vi "UHR-Fleezers Control (host) -Leonardo 04-2018 V4_fish.vi"(0 "Tab Green FB":T5(tab)=enum."Trap Control (RF)") -> ()   [LabVIEW 2014] (continued)
              }
            }
          }
          frame Enabled {
            n955 = call "hamilton_controller.vi"("Open?"=w1537, "valve"=enum16{"A", "B", "C", "D", "ALL"}."A", "action"=T21."MOVE VALVE") -> ()  [unwired: 8 in, 1 out]
          }
        }
      }
      event "Inject Valve B": Value Change {
        n956 = event-data() -> ()  [unwired: 7 out]
        n957 = disable-structure shown="Enabled" {
          disable-tunnel: "Inject Valve B" -> [w1541 w1561]
          frame Disabled {
            n958 = local read "Pump write delay (ms)"() -> (w1543:dbl)
            n959 = flat-sequence {
              tunnel: w1542 -> [w1556]
              tunnel: w1543 -> [w1552]
              tunnel: w1541 -> [_]
              tunnel: w1543 -> [w1558]
              tunnel: w1542 -> [w1559]
              frame #0 {
                n960 = local read "All Pump Parameters"() -> (w1551:T6)
                n961 = Multiply(x=60.0, y="Flush Center Ch Rate (ul/m)") -> (x*y=w1548:dbl)
                n962 = Unbundle By Name(w1551) -> ("Pump 2"=w1557:T33)
                n963 = call "Set pump parameters.vi"("Pump write delay (ms)"=w1552, "Volume (uL)"="Flush Center Ch Volume (uL)", "Rate (uL/h)"=w1548, "Units"=3.0, "Pump #"=2.0, "Pump Parameters In"=w1557, "VISA resource name"=w1556) -> ("Pump Parameters Out"=w1550:T33)  [unwired: 3 in]
                n964 = Bundle By Name(cluster=w1551, "Pump 2"=w1550) -> (w1549:T6)
                n965 = local write "All Pump Parameters"(w1549) -> ()
                n966 = Add(x="Flush Center Ch Volume (uL)", y="Total Volume\nFlushed (uL)") -> (x+y=w1545:dbl)
                n967 = local write "Total Volume\nFlushed (uL)"(w1545) -> ()
              }
              frame #1 {
                n968 = Wait (ms)(milliseconds to wait=w1558) -> ()  [unwired: 1 out]
              }
              frame #2 {
                n969 = call "Write to pump.vi"("string"="start", "VISA resource name"=w1559) -> ()  [unwired: 1 out]
              }
            }
            n970 = local read "Chemyx Syringe Pump Serial Port"() -> (w1542:refnum<visa-resource-name>)
          }
          frame Enabled {
            n971 = call "hamilton_controller.vi"("Open?"=w1561, "valve"=enum16{"A", "B", "C", "D", "ALL"}."B", "action"=T21."MOVE VALVE") -> ()  [unwired: 8 in, 1 out]
          }
        }
      }
      event "Inject Bottom": Value Change {
        n972 = event-data() -> ()  [unwired: 7 out]
        n973 = call "hamilton_controller.vi"("Open?"="Inject Bottom", "valve"=enum16{"A", "B", "C", "D", "ALL"}."C", "action"=T21."MOVE VALVE") -> ()  [unwired: 8 in, 1 out]
      }
      event "Shunt:": Value Change {
        n974 = event-data() -> ()  [unwired: 7 out]
        n975 = call "hamilton_controller.vi"("Open?"="Shunt:", "valve"=enum16{"A", "B", "C", "D", "ALL"}."D", "action"=T21."MOVE VALVE") -> ()  [unwired: 8 in, 1 out]
      }
      event "Flip Green Filter": Value Change {
        n976 = event-data() -> ()  [unwired: 7 out]
        n977 = local write "Flip Green Filter"("Flip Green Filter") -> ()
        n978 = flat-sequence {
          tunnel: w1577 -> [w1582]
          tunnel: w1576 -> [w1581]
          tunnel: [w1579] -> w1574
          tunnel: [w1578] -> w1573
          tunnel: [w1584] -> w1572
          tunnel: w1574 -> [w1584]
          tunnel: [w1583] -> w1571
          tunnel: w1573 -> [w1583]
          tunnel: w1572 -> [w1588]
          tunnel: w1571 -> [w1587]
          tunnel: [w1586] -> w1575
          frame #0 {
            n979 = xnode "Read/Write Control"("FPGA VI Reference In"=w1582, "error in"=w1581, "Green Filter Flipper"=TRUE) -> ("FPGA VI Reference Out"=w1579:T20, "error out"=w1578:errorcluster)
          }
          frame #1 {
            n980 = Wait (ms)(milliseconds to wait=u32 100) -> ()  [unwired: 1 out]
          }
          frame #2 {
            n981 = xnode "Read/Write Control"("FPGA VI Reference In"=w1588, "error in"=w1587, "Green Filter Flipper"=FALSE) -> ("error out"=w1586:errorcluster)  [unwired: 1 out]
          }
        }
      }
      event "Pump 1 contents", "Pump 3 contents": Value Change {
        n982 = event-data() -> ()  [unwired: 7 out]
        n983 = local read "Pump 1 contents"() -> (→"Pump 1 cont disp":string)
        n984 = local read "Pump 3 contents"() -> (→"Pump 3 cont disp":string)
      }
      event "Reset Trap Pos. FB": Value Change {
        n985 = event-data() -> ()  [unwired: 7 out]
        n986 = xnode "Read/Write Control"("FPGA VI Reference In"=w1594, "error in"=w1593, "Trap Pos. FB Reset"="Reset Trap Pos. FB") -> ()  [unwired: 2 out]
      }
      event "Trap Pos. FB ON": Value Change {
        n987 = event-data() -> ()  [unwired: 7 out]
        n988 = xnode "Read/Write Control"("FPGA VI Reference In"=w1609, "error in"=w1608) -> ("FPGA VI Reference Out"=w1606:T20, "BD1 Frequency Out 1"=w1603:u64)  [unwired: 1 out]
        n989 = To Double Precision Float(number=w1603) -> (double precision float=w1602:dbl)
        n990 = Multiply(x=49125000.0, y=6.0) -> (x*y=w1601:dbl)
        n991 = Multiply(x=w1602, y=w1601) -> (x*y=w1599:dbl)
        n992 = Scale By Power Of 2(n=-48, x=w1599) -> (x*2^n=w1598:dbl)
        n993 = Divide(x=w1598, y=1000000.0) -> (x/y=w1595:dbl)
        n994 = flat-sequence {
          tunnel: [w1612] -> w1607
          tunnel: w1606 -> [w1613]
          tunnel: w1603 -> [w1611]
          tunnel: "Trap Pos. FB ON" -> [w1610]
          tunnel: "Trap Pos. FB ON" -> [w1619]
          tunnel: w1607 -> [w1618]
          tunnel: "Trap Pos. FB ON" -> [w1621]
          tunnel: w1595 -> [w1620]
          frame #0 {
            n995 = case shown="False" w1610 {
              tunnel: w1613 -> [w1616 w1617]
              tunnel: [w1615 w1617] -> w1612
              tunnel: w1611 -> [w1614 _]
              frame False {
                n996 = xnode "Read/Write Control"("FPGA VI Reference In"=w1616, "BD 1 Frequency 1"=w1614) -> ("FPGA VI Reference Out"=w1615:T20)  [unwired: 1 in, 1 out]
              }
              frame True {
              }
            }
          }
          frame #1 {
            n997 = xnode "Read/Write Control"("FPGA VI Reference In"=w1618, "Force feedback"=w1619) -> ()  [unwired: 1 in, 2 out]
          }
          frame #2 {
            n998 = case shown="False" w1621 {
              tunnel: w1620 -> [w1624 _]
              frame False {
                n999 = local read "T2 for asymmetric\n(MHz)"() -> (w1622:dbl)
                n1000 = Subtract(x=w1622, y=w1624) -> (x-y=w1623:dbl)
                n1001 = property on="Trap Delta (MHz)" class="DigNum (strict)"("Val(Sgnl)"=w1623) -> ()  [unwired: 2 in, 2 out]
              }
              frame True {
              }
            }
          }
        }
      }
      event "Diff. FB.", "Trap Pos. FB Gains", "Trap Pos. FB Mult Factor", "Trap Pos. FB Offset Factor", "Trap Pos FB Negate Action", "Trap Pos FB Monitor\nT1 or T2", "Negate Diff?": Value Change {
        n1002 = event-data() -> ()  [unwired: 7 out]
        n1003 = xnode "Read/Write Control"("FPGA VI Reference In"=w1635, "error in"=w1634, "Trap pos. FB Range"="Trap Pos. FB Range", "Trap Pos. FB Gains"="Trap Pos. FB Gains", "Trap Pos. FB Mult Factor"="Trap Pos. FB Mult Factor", "Trap Pos. FB Offset Factor"="Trap Pos. FB Offset Factor", "Trap Pos FB Negate Action"="Trap Pos FB Negate Action", "Trap Pos FB Monitor T1 or T2"="Trap Pos FB Monitor\nT1 or T2", "AI1 X Scale"="Trap Pos. AI1 X Pre-scale", "Negate Diff?"="Negate Diff?", "Diff FB Measurement?"="Diff. FB.") -> ()  [unwired: 2 out]
      }
      event "Trap Pos FB SP": Value Change {
        n1004 = event-data() -> ()  [unwired: 7 out]
        n1005 = xnode "Read/Write Control"("FPGA VI Reference In"=w1638, "error in"=w1637, "Trap Pos. FB SP"="Trap Pos FB SP") -> ()  [unwired: 2 out]
        n1006 = disable-structure shown="Disabled" {
          frame Disabled {
            n1007 = local read "Trap X AI1 (DMA)"() -> (w1659:T13)
            n1008 = local read "Trap X (AI1)"() -> (w1660:T1)
            n1009 = local read "Setpoint offset\nCorrection values"() -> (w1653:dbl[])
            n1010 = local read "Trap Delta (MHz)"() -> (w1657:dbl)
            n1011 = local read "B factor"() -> (w1644:dbl)
            n1012 = Unbundle(w1660) -> ("Trap 1"=w1658:fxp<+/-,16,1>, "Trap 2"=w1647:fxp<+/-,16,1>)
            n1013 = Unbundle(w1659) -> ("Set 1"=w1643:fxp<+/-,16,1>, "Set 2"=w1642:fxp<+/-,16,1>)
            n1014 = Negate(x=w1647) -> (-x=w1640:fxp<+/-,17,2>)
            n1015 = Negate(x=w1658) -> (-x=w1641:fxp<+/-,17,2>)
            n1016 = Divide(x=w1657, y=0.1) -> (x/y=w1655:dbl)
            n1017 = Multiply(x=w1642, y=w1644) -> (x*y=w1645:dbl)
            n1018 = Subtract(x=w1643, y=w1645) -> (x-y=w1650:dbl)
            n1019 = To Long Integer(number=w1655) -> (32bit integer=w1654:i32)
            n1020 = Index Array(array=w1653, index=w1654) -> (element=w1649:dbl)
            n1021 = Multiply(x=w1644, y=w1640) -> (x*y=w1646:dbl)
            n1022 = Subtract(x=w1641, y=w1646) -> (x-y=w1652:dbl)
            n1023 = Add(x=w1652, y=w1649) -> (x+y=→"ideal setpoint fpga":dbl)
            n1024 = Add(x=w1650, y=w1649) -> (x+y=→"ideal setpoint avgd":dbl)
          }
          frame Enabled {
          }
        }
        n1025 = disable-structure shown="Enabled" {
          frame Enabled {
          }
          frame Disabled {
            n1026 = local write "B factor"(1.0 ("B factor")) -> ()
          }
        }
      }
      event "Simulate stepping": Value Change {
        n1027 = event-data() -> ()  [unwired: 7 out]
        n1028 = flat-sequence {
          tunnel: w1662 -> [w1665]
          tunnel: [w1664] -> _
          tunnel: w1661 -> [w1663]
          frame #0 {
            n1029 = while {
              tunnel: w1665 -> [w1693]
              tunnel: [w1692] -> w1664 mode=indexing
              tunnel: w1663 -> [w1691]
              i -> [w1677]
              stop <- w1674 stop-if-true
              w1667 = 1000.0
              n1030 = Divide(x="Backtrack probability", y=100) -> (x/y=w1701:dbl)
              n1031 = Random Number (0-1)() -> (number: 0 to 1=w1702:dbl)
              n1032 = Greater?(x=w1702, y=w1701) -> (0:w1700:bool)
              n1033 = Select(t=1, s=w1700, f=-1) -> (s? t:f=w1697:i32)
              n1034 = local read "BD 1 Frequency 2 (MHz)"() -> (w1672:dbl)
              n1035 = Multiply(x=w1697, y="Step size (nm)") -> (x*y=w1695:dbl)
              "Step taken" <- w1695
              n1036 = Divide(x=w1695, y=168.33) -> (x/y=w1670:dbl)
              n1037 = local read "BD 1 Frequency 1 (MHz)"() -> (w1671:dbl)
              n1038 = local read "X RF Frequency Limits (MHz)"() -> (w1690:T16)
              n1039 = local read "Y RF Frequency Limits (MHz)"() -> (w1689:T16)
              n1040 = Subtract(x=w1671, y=w1670) -> (x-y=w1669:dbl)
              n1041 = local write "BD 1 Frequency 1 (MHz)"(w1669) -> ()
              n1042 = local read "BD 2 Frequency 1 (MHz)"() -> (w1687:dbl)
              n1043 = local read "BD 2 Frequency 2 (MHz)"() -> (w1688:dbl)
              n1044 = call "set RF board frequency - interlace.vi"("Board 2 Frequency Limits"=w1689, "Board 1 Frequency Limits"=w1690, "error in"=w1693, "FPGA VI Reference In"=w1691, "Board 2 Frequency 2 (MHz)"=w1688, "Board 2 Frequency 1 (MHz)"=w1687, "Board 1 Frequency 2 (MHz)"=w1672, "Board 1 Frequency 1  (MHz)"=w1669) -> ("error out"=w1692:errorcluster)  [unwired: 2 in, 1 out]
              n1045 = Subtract(x=w1672, y=w1669) -> (x-y=w1686:dbl)
              n1046 = Subtract(x=w1688, y=w1687) -> (x-y=w1685:dbl)
              n1047 = Square(x=w1685) -> (x^2=w1683:dbl)
              n1048 = Square(x=w1686) -> (x^2=w1684:dbl)
              n1049 = Add(x=w1684, y=w1683) -> (x+y=w1682:dbl)
              n1050 = Square Root(x=w1682) -> (sqrt(x)=w1673:dbl)
              n1051 = local write "Trap Delta (MHz)"(w1673) -> ()
              n1052 = property on="Initial delta (MHz)" class="DigNum (strict)"("Val(Sgnl)"=w1673) -> ()  [unwired: 2 in, 2 out]
              n1053 = Multiply(x="Mean dwell time (s)", y=w1667) -> (x*y=w1679:dbl)
              n1054 = case shown="\"Gamma2\"" "Distribution" {
                tunnel: w1679 -> [w1706 w1710 w1713]
                tunnel: [w1706 w1707 w1714] -> w1668
                frame "uniform", Default {
                }
                frame "Exponential" {
                  n1055 = call-poly <vilib>:"Continuous Random.vi"("b"=w1710, "samples"=1) -> ("exp random data"=w1708:dbl[])  [unwired: 8 in, 1 out]
                  n1056 = Index Array(array=w1708) -> (element=w1707:dbl)  [unwired: 1 in]
                }
                frame "Gamma2" {
                  w1711 = 2.0
                  # "Note: the shape and scale\nparameters of the gamma\nare inverted because LabView..."
                  n1057 = Divide(x=w1713, y=w1711) -> (x/y=w1712:dbl)
                  n1058 = call-poly <vilib>:"Continuous Random.vi"("c"=w1712, "b"=w1711, "samples"=1) -> ("gamma random numbers"=w1715:dbl[])  [unwired: 7 in, 1 out]
                  n1059 = Index Array(array=w1715) -> (element=w1714:dbl)  [unwired: 1 in]
                }
              }
              n1060 = Divide(x=w1668, y=w1667) -> (x/y=→"Step duration":dbl)
              n1061 = To Unsigned Long Integer(number=w1668) -> (unsigned 32bit integer=w1680:u32)
              n1062 = Add(x=w1677, y=1) -> (x+y=w1676:i32)
              n1063 = Wait (ms)(milliseconds to wait=w1680) -> ()  [unwired: 1 out]
              n1064 = Equal?(x=w1676, y="Number of steps") -> (x = y?=w1674:bool)
            }
          }
          frame #1 {
            n1065 = local write "Simulate stepping"(FALSE) -> ()
          }
        }
      }
      event "Set SP to Reading": Value Change {
        n1066 = event-data() -> ()  [unwired: 7 out]
        n1067 = local read "Trap Pos FB Monitor\nT1 or T2"() -> (w1725:bool)
        n1068 = local read "Trap X AI1 (DMA)"() -> (w1728:T13)
        n1069 = local read "Trap X (AI1)"() -> (w1731:T1)
        n1070 = Unbundle By Name(w1731) -> ("Trap 1"=w1730:fxp<+/-,16,1>, "Trap 2"=w1729:fxp<+/-,16,1>)
        n1071 = Unbundle By Name(w1728) -> ("Set 1"=w1727:fxp<+/-,16,1>, "Set 2"=w1726:fxp<+/-,16,1>)
        n1072 = Select(t=w1730, s=w1725, f=w1729) -> (s? t:f=w1724:fxp<+/-,16,1>)
        n1073 = Select(t=w1727, s=w1725, f=w1726) -> (s? t:f=w1723:fxp<+/-,16,1>)
        n1074 = Not(x="Set SP Using...") -> (.not. x?=w1718:bool)
        n1075 = Select(t=w1724, s=w1718, f=w1723) -> (s? t:f=w1719:fxp<+/-,16,1>)
        n1076 = xnode "Read/Write Control"("FPGA VI Reference In"=w1721, "error in"=w1720, "Trap Pos. FB SP"=w1719) -> ()  [unwired: 2 out]
        n1077 = local write "Trap Pos FB SP"(w1719) -> ()
      }
      event "Trap Pos. FB Out Scale 2^n": Value Change {
        n1078 = event-data() -> ()  [unwired: 7 out]
        n1079 = Scale By Power Of 2(n="Trap Pos. FB Out Scale 2^n", x=ext 1.0) -> (x*2^n=w1733:ext)
        n1080 = property on="Trap Pos. FB Mult Factor" class="DigNum (strict)"("Val(Sgnl)"=w1733) -> ()  [unwired: 2 in, 2 out]
      }
      event "Trap Pos FB Int Count": Value Change {
        n1081 = event-data() -> ()  [unwired: 7 out]
        n1082 = xnode "Read/Write Control"("FPGA VI Reference In"=w1738, "error in"=w1737, "Trap Pos FB Int Count"="Trap Pos FB Int Count") -> ()  [unwired: 2 out]
      }
      event "Target Force (pN)", "Setpoint offset\nCorrection values", "Raster target force (pN)": Value Change {
        w1747 = 2.0
        n1083 = event-data() -> ()  [unwired: 7 out]
        n1084 = disable-structure "Removed B Factor to improve position feedback - Alex 081418 1of3" shown="Enabled" {
          disable-tunnel: [w1777 fxp<+/-,32,16> 1.0 ("B factor")] -> w1739
          frame Disabled {
            n1085 = local read "B factor"() -> (w1778:dbl)
            n1086 = To Fixed-Point(number=w1778) -> (fixed-point=w1777:fxp<+/-,16,16>)  [unwired: 1 in]
          }
          frame Enabled {
          }
        }
        n1087 = xnode "Read/Write Control"("FPGA VI Reference In"=w1741, "B factor"=w1739) -> ("BD1 Frequency Out 1"=w1768:u64)  [unwired: 1 in, 2 out]
        n1088 = local read "BD 1 Frequency 2 (MHz)"() -> (w1767:dbl)
        n1089 = local read "Target Force (pN)"() -> (w1753:dbl)
        n1090 = To Double Precision Float(number=w1768) -> (double precision float=w1774:dbl)
        n1091 = Multiply(x=49125000.0, y=6.0) -> (x*y=w1773:dbl)
        n1092 = Multiply(x=w1774, y=w1773) -> (x*y=w1771:dbl)
        n1093 = Scale By Power Of 2(n=-48, x=w1771) -> (x*2^n=w1770:dbl)
        n1094 = Divide(x=w1770, y=1000000.0) -> (x/y=w1766:dbl)
        n1095 = Subtract(x=w1767, y=w1766) -> (x-y=w1765:dbl)
        n1096 = local read "T1 kappa_x (pN/nm)"() -> (w1754:dbl)
        n1097 = local read "T1 alpha_x (nm/V)"() -> (w1755:dbl)
        n1098 = local read "Negate offset difference"() -> (w1756:bool)
        n1099 = local read "Offset file step size"() -> (w1764:dbl)
        n1100 = Multiply(x="Raster target force (pN)", y=w1747) -> (x*y=w1746:dbl)
        n1101 = Multiply(x=w1753, y=w1747) -> (x*y=w1752:dbl)
        n1102 = local read "Setpoint offset\nCorrection values"() -> (w1761:dbl[])
        n1103 = Divide(x=w1765, y=w1764) -> (x/y=w1763:dbl)
        n1104 = Select(t=-1, s=w1756, f=1) -> (s? t:f=w1757:i32)
        n1105 = To Long Integer(number=w1763) -> (32bit integer=w1762:i32)
        n1106 = Multiply(x=w1755, y=w1754) -> (x*y=w1745:dbl)
        n1107 = Divide(x=w1752, y=w1745) -> (x/y=w1751:dbl)
        n1108 = Index Array(array=w1761, index=w1762) -> (element=w1760:dbl)
        n1109 = Divide(x=w1746, y=w1745) -> (x/y=w1744:dbl)
        n1110 = Multiply(x=w1757, y=w1760) -> (x*y=w1743:dbl)
        n1111 = Add(x=w1751, y=w1743) -> (x+y=w1750:dbl)
        n1112 = Add(x=w1744, y=w1743) -> (x+y=w1742:dbl)
        n1113 = To Fixed-Point(number=w1742) -> (fixed-point=w1740:fxp<+/-,16,1>)  [unwired: 1 in]
        n1114 = To Fixed-Point(number=w1750) -> (fixed-point=w1749:fxp<+/-,16,1>)  [unwired: 1 in]
        n1115 = property on="Trap Pos FB SP" class="DigNum (strict)"("Val(Sgnl)"=w1749) -> ()  [unwired: 2 in, 2 out]
        n1116 = xnode "Read/Write Control"("FPGA VI Reference In"=w1741, "Raster setpoint"=w1740) -> ()  [unwired: 1 in, 2 out]
      }
      event "Read setpoint correction\nfile": Value Change {
        n1117 = event-data() -> ()  [unwired: 7 out]
        n1118 = local write "Read setpoint correction\nfile"(FALSE) -> ()
        n1119 = Open/Create/Replace File(file path (use dialog)="Setpoint correction\noffset file", operation (0:open)=T24."open", access (0:read/write)=enum16{"read/write", "read-only", "write-only"}."read-only") -> (refnum out=w1805:refnum<file>)  [unwired: 1 in, 4 out]
        n1120 = Deny Access(7:w1805) -> (3:w1803:refnum<file>)  [unwired: 1 in, 2 out]
        n1121 = Read from Binary File(5:0.0, 9:T30."big-endian, network order" ("byte order (0:big-endian, network order)"), 10:-1 ("count (1)"), 11:w1803) -> (2:w1796:dbl[], 3:w1802:refnum<file>)  [unwired: 1 in, 3 out]
        n1122 = Close File(refnum=w1802) -> ()  [unwired: 1 in, 2 out]
        n1123 = Index Array(array=w1796, index=0) -> (element=w1792:dbl)
        n1124 = local write "Offset file step size"(w1792) -> ()
        n1125 = Array Subset(array=w1796, index=3) -> (w1795:dbl[])  [unwired: 1 in]
        n1126 = local read "T1 kappa_x (pN/nm)"() -> (w1790:dbl)
        n1127 = local read "T1 alpha_x (nm/V)"() -> (w1791:dbl)
        n1128 = local read "T2 alpha_x (nm/V)"() -> (w1789:dbl)
        n1129 = local read "T2 kappa_x (pN/nm)"() -> (w1788:dbl)
        n1130 = Decimate 1D Array(w1795) -> (w1784:dbl[], w1785:dbl[])  [unwired: 1 out]
        n1131 = local read "Offset Values"() -> (w1794:T14)
        n1132 = Multiply(x=w1791, y=w1790) -> (x*y=w1786:dbl)
        n1133 = Multiply(x=w1789, y=w1788) -> (x*y=w1787:dbl)
        n1134 = Bundle By Name(cluster=w1794, "Trap 1X offset"=w1784, "Trap 2X offset"=w1785) -> (w1793:T14)
        n1135 = Divide(x=w1787, y=w1786) -> (x/y=w1781:dbl)
        n1136 = disable-structure "Removed B Factor to better position FB - Alex 081418 3of3" shown="Enabled" {
          disable-tunnel: w1781 -> [w1809 _]
          disable-tunnel: [w1809 1.0] -> w1780
          frame Disabled {
          }
          frame Enabled {
          }
        }
        n1137 = Multiply(x=w1785, y=w1780) -> (x*y=w1783:dbl[])
        n1138 = local write "Offset Values"(w1793) -> ()
        n1139 = Subtract(x=w1784, y=w1783) -> (x-y=w1782:dbl[])
        n1140 = property on="B factor" class="DigNum (strict)"("Val(Sgnl)"=w1780) -> ()  [unwired: 2 in, 2 out]
        n1141 = property on="Setpoint offset\nCorrection values" class="Arr (strict)"("Val(Sgnl)"=w1782) -> ()  [unwired: 2 in, 2 out]
      }
      event "MCL Tracking": Value Change {
        n1142 = event-data() -> ()  [unwired: 7 out]
        n1143 = case shown="True" "MCL Tracking" {
          frame False {
            n1144 = local read "Current MCL (V)"() -> (w1812:dbl)
            n1145 = local write "AO2"(w1812) -> ()
          }
          frame True {
            n1146 = local read "BD 1 Frequency 1 (MHz)"() -> (→"Zero T1 position":dbl)
            n1147 = local read "AO2"() -> (→"Zero MCL x position":dbl)
          }
        }
      }
      event "Scale intensities": Value Change {
        n1148 = event-data() -> ()  [unwired: 7 out]
        n1149 = local read "Trap Intensity\nSetpoints (V)"() -> (w1818:cluster{"Set 1":dbl, "Set 2":dbl})
        n1150 = local read "T1 kappa_x (pN/nm)"() -> (w1824:dbl)
        n1151 = local read "T2 kappa_x (pN/nm)"() -> (w1823:dbl)
        n1152 = Unbundle By Name(w1818) -> ("Set 1"=w1820:dbl, "Set 2"=w1819:dbl)
        n1153 = case shown="True" "Scale intensities" {
          tunnel: "Scale factor" -> [w1834 w1846]
          tunnel: "Scale factor" -> [w1829 w1839]
          tunnel: w1824 -> [w1836 w1845]
          tunnel: w1823 -> [w1835 w1844]
          tunnel: [w1832 w1843] -> w1822
          tunnel: [w1833 w1842] -> w1821
          tunnel: w1820 -> [w1831 w1841]
          tunnel: w1819 -> [w1830 w1840]
          tunnel: [w1828 w1838] -> w1817
          tunnel: [w1827 w1837] -> w1816
          frame False {
            n1154 = Divide(x=w1836, y=w1829) -> (x/y=w1832:dbl)
            n1155 = Divide(x=w1835, y=w1834) -> (x/y=w1833:dbl)
            n1156 = Divide(x=w1831, y=w1829) -> (x/y=w1828:dbl)
            n1157 = Divide(x=w1830, y=w1829) -> (x/y=w1827:dbl)
          }
          frame True {
            n1158 = Multiply(x=w1841, y=w1839) -> (x*y=w1838:dbl)
            n1159 = Multiply(x=w1840, y=w1839) -> (x*y=w1837:dbl)
            n1160 = Multiply(x=w1845, y=w1839) -> (x*y=w1843:dbl)
            n1161 = Multiply(x=w1846, y=w1844) -> (x*y=w1842:dbl)
          }
        }
        n1162 = local write "T2 kappa_x (pN/nm)"(w1821) -> ()
        n1163 = local write "T1 kappa_x (pN/nm)"(w1822) -> ()
        n1164 = Bundle By Name(cluster=w1818, "Set 1"=w1817, "Set 2"=w1816) -> (w1815:cluster{"Set 1":dbl, "Set 2":dbl})
        n1165 = property on="Trap Intensity\nSetpoints (V)" class="Clust (strict)"("Val(Sgnl)"=w1815) -> ()  [unwired: 2 in, 2 out]
      }
    }
    "error out 2" <- w773
    n1166 = node-c288() -> ()  [unwired: 1 in, 1 out]
  }
  n1167 = node-c288() -> (w104:T25)  [unwired: 4 in]
  n1168 = timed-loop "Run Scripts, including: stage motion" {
    timing: w104 -> [_]
    timing-out: [_] -> w103
    tunnel: w62 -> [_]
    stop <- w1848 stop-if-true
    n1169 = node-c288() -> ()  [unwired: 1 in, 1 out]
    n1170 = event shown="[0] \"Move Cap. 1 (DNA Top)\": Value Change" {
      selector: _ -> [_ _ _ _ _ _ _ _ _ _ _ _]
      dyn-events: _ -> [_ _ _ _ _ _ _ _ _ _ _ _]
      timeout: 50 -> [_ _ _ _ _ _ _ _ _ _ _ _]
      tunnel: ["Move Cap. 1 (DNA Top)" _ "Cal/Data Acq. Spot" "Dump Beads" "Dip for Protein" _ "Got ADig bead" "Got DNA bead" "Take Stepping Data" _ "Take Detection Laser\nImage" _] -> _
      tunnel: [_ _ _ _ _ _ _ _ _ _ _ w2058] -> w1848
      event "Move Cap. 1 (DNA Top)": Value Change {
        n1171 = event-data() -> ()  [unwired: 1 in, 5 out]
        n1172 = local write "Move Cap. 1 (DNA Top)"(FALSE ("Move Cap. 1 (DNA Right)")) -> ()
        n1173 = flat-sequence {
          tunnel: "Cap 1 Samp Flow ON" -> [w1854]
          frame #0 {
            n1174 = local write "Stage Moving"(FALSE ("Stage Moving")) -> ()
            n1175 = case "stop flow" shown="True" w1854 {
              frame False {
              }
              frame True {
                n1176 = call "hamilton_controller.vi"("Open?"=FALSE, "valve"=enum16{"A", "B", "C", "D", "ALL"}."C", "action"=T21."MOVE VALVE") -> ()  [unwired: 8 in, 1 out]
              }
            }
            n1177 = case shown="True" TRUE {
              tunnel: "Cap 1 T ON" -> [w1863 w1864]
              frame False {
                n1178 = property on="Trap 1 (ON/OFF)" class="Bool (strict)"("Val(Sgnl)"=w1863) -> ()  [unwired: 2 in, 2 out]
              }
              frame True {
                n1179 = property on="Trap 2 (ON/OFF)" class="Bool (strict)"("Val(Sgnl)"=w1864) -> ()  [unwired: 2 in, 2 out]
              }
            }
            n1180 = call <vilib>:"Beep.vi"() -> ()  [unwired: 3 in, 9 out]
            n1181 = case shown="True" "Cap 1 Flow ON" {
              frame False {
              }
              frame True {
                n1182 = property on="Main:" class="Bool (strict)"("Val(Sgnl)"=TRUE ("Value (Signaling)")) -> ()  [unwired: 2 in, 2 out]
              }
            }
          }
        }
      }
      event Timeout {
        n1183 = event-data() -> ()  [unwired: 1 in, 2 out]
      }
      event "Cal/Data Acq. Spot": Value Change {
        # "wait for calibration file\nto be written"
        # "signal save cal true\nthis tells the data \nacquisition loop to\nstart sending the data\nto a calibration file"
        # "separate traps to\nthe desired trap delta"
        # "move stage to data acquisition spot"
        # "CHANGE FISH FOR TETHER BACK\nTO TRUE VALUE HERE."
        n1184 = event-data() -> ()  [unwired: 1 in, 5 out]
        n1185 = flat-sequence {
          tunnel: ["Cal @ (MHz)"] -> w1865
          tunnel: w1865 -> [w1877]
          tunnel: w1865 -> [w1898]
          frame #0 {
            n1186 = property on="Trap Delta (MHz)" class="DigNum (strict)"("Val(Sgnl)"="Cal @ (MHz)") -> ()  [unwired: 2 in, 2 out]
            n1187 = call <vilib>:"Beep.vi"() -> ()  [unwired: 3 in, 9 out]
          }
          frame #1 {
            n1188 = local read "Scale intensities"() -> (w1869:bool)
            n1189 = case shown="True" w1869 {
              frame False {
              }
              frame True {
                n1190 = property on="Scale intensities" class="Bool (strict)"("Val(Sgnl)"=FALSE ("Value (Signaling)")) -> ()  [unwired: 2 in, 2 out]
              }
            }
          }
          frame #2 {
            n1191 = Wait (ms)(milliseconds to wait=u32 500) -> ()  [unwired: 1 out]
          }
          frame #3 {
            n1192 = property on="Save Calibration" class="Bool (strict)"("Val(Sgnl)"=TRUE ("Value (Signaling)")) -> ()  [unwired: 2 in, 2 out]
          }
          frame #4 {
            n1193 = Wait (ms)(milliseconds to wait=u32 4000) -> ()  [unwired: 1 out]
          }
          frame #5 {
            n1194 = while {
              stop <- w1874 stop-if-true
              n1195 = local read "Saving..."() -> (w1875:bool)
              n1196 = Wait (ms)(milliseconds to wait=u32 100) -> ()  [unwired: 1 out]
              n1197 = Not(x=w1875) -> (.not. x?=w1874:bool)
            }
          }
          frame #6 {
            n1198 = case shown="True" "W/ Offset 1" {
              tunnel: w1877 -> [_ w1879]
              frame False {
              }
              frame True {
                n1199 = stacked-sequence {
                  tunnel: w1879 -> [_ _ _ _ _ _ _ w1896]
                  frame #0 {
                    n1200 = Replace Array Subset(array=u32[] [0] ("Index Values"), new element="Offset 1 Set", index=0) -> (w1880:u32[])
                    n1201 = property on="Saved AOD Raster Scan Parameter Sets" class="Arr (strict)"("Index Values"=w1880) -> ()  [unwired: 2 in, 2 out]
                    n1202 = property on="Trap Delta (MHz)" class="DigNum (strict)"("Val(Sgnl)"="Offset 1 Start (MHz)") -> ()  [unwired: 2 in, 2 out]
                  }
                  frame #1 {
                    n1203 = Wait (ms)(milliseconds to wait=u32 200) -> ()  [unwired: 1 out]
                  }
                  frame #2 {
                    n1204 = property on="Load parameters" class="Bool (strict)"("Val(Sgnl)"=TRUE ("Value (Signaling)")) -> ()  [unwired: 2 in, 2 out]
                  }
                  frame #3 {
                    n1205 = Wait (ms)(milliseconds to wait=u32 200) -> ()  [unwired: 1 out]
                  }
                  frame #4 {
                    n1206 = property on="Trap Raster Scan" class="Bool (strict)"("Val(Sgnl)"=TRUE ("Value (Signaling)")) -> ()  [unwired: 2 in, 2 out]
                  }
                  frame #5 {
                    n1207 = Wait (ms)(milliseconds to wait=u32 2000) -> ()  [unwired: 1 out]
                  }
                  frame #6 {
                    n1208 = while {
                      stop <- w1893 stop-if-true
                      n1209 = local read "Raster Scanning..."() -> (w1895:bool)
                      n1210 = local read "Saving..."() -> (w1891:bool)
                      n1211 = Wait (ms)(milliseconds to wait=u32 100) -> ()  [unwired: 1 out]
                      n1212 = Not(x=w1891) -> (.not. x?=w1890:bool)
                      n1213 = Not(x=w1895) -> (.not. x?=w1892:bool)
                      n1214 = And(x=w1892, y=w1890) -> (x .and. y?=w1893:bool)
                    }
                  }
                  frame #7 {
                    n1215 = property on="Trap Delta (MHz)" class="DigNum (strict)"("Val(Sgnl)"=w1896) -> ()  [unwired: 2 in, 2 out]
                  }
                }
              }
            }
          }
          frame #7 {
            n1216 = local read "Save ave N"() -> (w1897:dbl)
            n1217 = case shown="True" "W/ Offset 2" {
              tunnel: w1898 -> [_ w1904]
              tunnel: w1897 -> [_ w1903]
              frame False {
                n1218 = Multiply(x="Cal read wait (s)", y=u32 1000 ("milliseconds to wait")) -> (x*y=w1901:u32)
                n1219 = Wait (ms)(milliseconds to wait=w1901) -> ()  [unwired: 1 out]
              }
              frame True {
                n1220 = stacked-sequence {
                  tunnel: w1904 -> [_ _ _ _ _ _ _ _ _ w1925 _ _]
                  tunnel: w1903 -> [_ _ _ _ _ _ _ _ _ w1923 _ _]
                  frame #0 {
                    n1221 = property on="Save ave N" class="DigNum (strict)"("Val(Sgnl)"=1.0 ("Value (Signaling)")) -> ()  [unwired: 2 in, 2 out]
                  }
                  frame #1 {
                    n1222 = Wait (ms)(milliseconds to wait=u32 500) -> ()  [unwired: 1 out]
                  }
                  frame #2 {
                    n1223 = property on="Trap Delta (MHz)" class="DigNum (strict)"("Val(Sgnl)"="Offset 2 Start (MHz)") -> ()  [unwired: 2 in, 2 out]
                    n1224 = Replace Array Subset(array=u32[] [0] ("Index Values"), new element="Offset 2 Set", index=0) -> (w1909:u32[])
                    n1225 = property on="Saved AOD Raster Scan Parameter Sets" class="Arr (strict)"("Index Values"=w1909) -> ()  [unwired: 2 in, 2 out]
                  }
                  frame #3 {
                    n1226 = Wait (ms)(milliseconds to wait=u32 500) -> ()  [unwired: 1 out]
                  }
                  frame #4 {
                    n1227 = property on="Load parameters" class="Bool (strict)"("Val(Sgnl)"=TRUE ("Value (Signaling)")) -> ()  [unwired: 2 in, 2 out]
                  }
                  frame #5 {
                    n1228 = Wait (ms)(milliseconds to wait=u32 500) -> ()  [unwired: 1 out]
                  }
                  frame #6 {
                    n1229 = property on="Trap Raster Scan" class="Bool (strict)"("Val(Sgnl)"=TRUE ("Value (Signaling)")) -> ()  [unwired: 2 in, 2 out]
                  }
                  frame #7 {
                    n1230 = Wait (ms)(milliseconds to wait=u32 2000) -> ()  [unwired: 1 out]
                  }
                  frame #8 {
                    n1231 = while {
                      stop <- w1918 stop-if-true
                      n1232 = local read "Raster Scanning..."() -> (w1921:bool)
                      n1233 = local read "Saving..."() -> (w1919:bool)
                      n1234 = Wait (ms)(milliseconds to wait=u32 100) -> ()  [unwired: 1 out]
                      n1235 = Not(x=w1919) -> (.not. x?=w1917:bool)
                      n1236 = Not(x=w1921) -> (.not. x?=w1920:bool)
                      n1237 = And(x=w1920, y=w1917) -> (x .and. y?=w1918:bool)
                    }
                  }
                  frame #9 {
                    n1238 = property on="Trap Delta (MHz)" class="DigNum (strict)"("Val(Sgnl)"=w1925) -> ()  [unwired: 2 in, 2 out]
                    n1239 = property on="Saved AOD Raster Scan Parameter Sets" class="Arr (strict)"("Index Values"=u32[] [0]) -> ()  [unwired: 2 in, 2 out]
                    n1240 = property on="Save ave N" class="DigNum (strict)"("Val(Sgnl)"=w1923) -> ()  [unwired: 2 in, 2 out]
                  }
                  frame #10 {
                    n1241 = Wait (ms)(milliseconds to wait=u32 500) -> ()  [unwired: 1 out]
                  }
                  frame #11 {
                    n1242 = property on="Load parameters" class="Bool (strict)"("Val(Sgnl)"=TRUE ("Value (Signaling)")) -> ()  [unwired: 2 in, 2 out]
                  }
                }
              }
            }
          }
          frame #8 {
            n1243 = property on="Read Cal" class="Bool (strict)"("Val(Sgnl)"=TRUE ("Value (Signaling)")) -> ()  [unwired: 2 in, 2 out]
          }
          frame #9 {
            n1244 = Wait (ms)(milliseconds to wait=u32 500) -> ()  [unwired: 1 out]
          }
          frame #10 {
            n1245 = property on="Fish for Tether" class="Bool (strict)"("Val(Sgnl)"=FALSE ("Value (Signaling)")) -> ()  [unwired: 2 in, 2 out]
          }
        }
        n1246 = local write "Cal/Data Acq. Spot"(FALSE ("Cal/Data Acq. Spot")) -> ()
      }
      event "Dump Beads": Value Change {
        # "SCRIPT TO REMOVE BOTH BEADS FROM THE TRAPS. TURNS ON LIGHT WHICH INDICATES THAT STAGE IS MOVING. THEN STOPS SAVING DATA. \nSETS Sample Channel Flow TO TRUE. STOPS INTERLACING GREEN FLUORESCENCE. TURNS OFF Tether INDICATOR BECAUSE WE ARE THROWING IT\nAWAY. SHUTS OFF TRAP POSITION FEEDBACK."
        n1247 = event-data() -> ()  [unwired: 1 in, 5 out]
        n1248 = flat-sequence {
          frame #0 {
            w1932 = FALSE ("Fl. Triggered...")
            w1933 = TRUE ("Stage Moving")
            n1249 = local read "Saving..."() -> (w1934:bool)
            n1250 = local write "Fl. Triggered..."(w1932) -> ()
            n1251 = local write "Stage Moving"(w1933) -> ()
            n1252 = local write "Tether"(w1932) -> ()
            n1253 = property on="Green Laser ON/Interlacing" class="Bool (strict)"("Val(Sgnl)"=w1932) -> ()  [unwired: 2 in, 2 out]
            n1254 = property on="Trap Pos. FB ON" class="Bool (strict)"("Val(Sgnl)"=w1932) -> ()  [unwired: 2 in, 2 out]
            n1255 = property on="Inject Bottom" class="Bool (strict)"("Val(Sgnl)"=w1933) -> ()  [unwired: 2 in, 2 out]
            n1256 = local write "Stop Saving"(w1934) -> ()
          }
          frame #1 {
            w1935 = FALSE ("Value (Signaling)")
            # "TURNS TRAPS OFF SO THAT\nBEADS REMAIN AT DUMP \nBEADS POSITION"
            n1257 = property on="Trap 1 (ON/OFF)" class="Bool (strict)"("Val(Sgnl)"=w1935) -> ()  [unwired: 2 in, 2 out]
            n1258 = property on="Trap 2 (ON/OFF)" class="Bool (strict)"("Val(Sgnl)"=w1935) -> ()  [unwired: 2 in, 2 out]
            n1259 = call <vilib>:"Beep.vi"() -> ()  [unwired: 3 in, 9 out]
          }
          frame #2 {
            n1260 = property on="Goto Bottom (F7)" class="Bool"("Val(Sgnl)"=TRUE ("Value (Signaling)")) -> ()  [unwired: 2 in, 2 out]
          }
          frame #3 {
            n1261 = Wait (ms)(milliseconds to wait=u32 8000) -> ()  [unwired: 1 out]
          }
          frame #4 {
            n1262 = property on="Trap Delta (MHz)" class="DigNum (strict)"("Val(Sgnl)"=20.0 ("Value (Signaling)")) -> ()  [unwired: 2 in, 2 out]
          }
          frame #5 {
            n1263 = property on="Trap 2 (ON/OFF)" class="Bool (strict)"("Val(Sgnl)"=TRUE ("Value (Signaling)")) -> ()  [unwired: 2 in, 2 out]
          }
          frame #6 {
            n1264 = property on="Inject Bottom" class="Bool (strict)"("Val(Sgnl)"=FALSE ("Value (Signaling)")) -> ()  [unwired: 2 in, 2 out]
          }
        }
      }
      event "Dip for Protein": Value Change {
        n1265 = event-data() -> ()  [unwired: 1 in, 5 out]
        n1266 = flat-sequence {
          frame #0 {
            n1267 = case shown="True" "Move Trap Before?" {
              frame False {
              }
              frame True {
                n1268 = property on="Trap Delta (MHz)" class="DigNum (strict)"("Val(Sgnl)"="Dip Trap Delta 1 (MHz)") -> ()  [unwired: 2 in, 2 out]
              }
            }
          }
          frame #1 {
            n1269 = Multiply(x="Duration (s)", y=1000.0) -> (x*y=w1944:dbl)
            n1270 = Wait (ms)(milliseconds to wait=w1944) -> ()  [unwired: 1 out]
          }
          frame #2 {
            n1271 = case shown="True" "Move Trap After?" {
              frame False {
              }
              frame True {
                n1272 = property on="Trap Delta (MHz)" class="DigNum (strict)"("Val(Sgnl)"="Dip Trap Delta 2 (MHz)") -> ()  [unwired: 2 in, 2 out]
              }
            }
          }
          frame #3 {
            n1273 = case shown="True" "Green ON After?" {
              frame False {
              }
              frame True {
                n1274 = property on="Green Laser ON/Interlacing" class="Bool (strict)"("Val(Sgnl)"=TRUE ("Value (Signaling)")) -> ()  [unwired: 2 in, 2 out]
              }
            }
          }
          frame #4 {
            n1275 = Wait (ms)(milliseconds to wait=u32 500) -> ()  [unwired: 1 out]
          }
          frame #5 {
            n1276 = case shown="True" "Save Data After?" {
              frame False {
              }
              frame True {
                n1277 = property on="Start Saving" class="Bool (strict)"("Val(Sgnl)"=TRUE ("Value (Signaling)")) -> ()  [unwired: 2 in, 2 out]
              }
            }
          }
        }
      }
      event "Profile": Value Change {
        n1278 = event-data() -> ()  [unwired: 1 in, 5 out]
        n1279 = flat-sequence {
          frame #0 {
            w1954 = 0.0 ("element")
            n1280 = Build Array(w1954, "Y change (mm)", w1954) -> ()  [unwired: 1 out]
          }
          frame #1 {
            # "stop saving"
            n1281 = local write "Stop Saving"(TRUE ("Stop Saving")) -> ()
            n1282 = local write "Stage Moving"(FALSE ("Stage Moving")) -> ()
          }
        }
      }
      event "Got ADig bead": Value Change {
        n1283 = event-data() -> ()  [unwired: 1 in, 5 out]
        n1284 = property on="Move Cap. 1 (DNA Top)" class="Bool (strict)"("Val(Sgnl)"=TRUE ("Value (Signaling)")) -> ()  [unwired: 2 in, 2 out]
        n1285 = property on="Inject Top:" class="Bool (strict)"("Val(Sgnl)"=FALSE ("Value (Signaling)")) -> ()  [unwired: 2 in, 2 out]
      }
      event "Got DNA bead": Value Change {
        n1286 = event-data() -> ()  [unwired: 1 in, 5 out]
        n1287 = property on="Cal/Data Acq. Spot" class="Bool (strict)"("Val(Sgnl)"=TRUE ("Value (Signaling)")) -> ()  [unwired: 2 in, 2 out]
        n1288 = property on="Main:" class="Bool (strict)"("Val(Sgnl)"=FALSE ("Value (Signaling)")) -> ()  [unwired: 2 in, 2 out]
      }
      event "Take Stepping Data": Value Change {
        n1289 = event-data() -> ()  [unwired: 1 in, 5 out]
        n1290 = local read "Save ave N"() -> (w1972:dbl)
        n1291 = flat-sequence {
          tunnel: w1972 -> [w1974]
          tunnel: [w1974] -> w1967
          tunnel: [w1976] -> w1968
          tunnel: w1967 -> [w1976]
          tunnel: [w1978] -> w1969
          tunnel: w1968 -> [w1978]
          tunnel: [w1981] -> w1970
          tunnel: w1969 -> [w1981]
          tunnel: [w1983] -> w1971
          tunnel: w1970 -> [w1983]
          tunnel: [w1985] -> w1965
          tunnel: w1971 -> [w1985]
          tunnel: w1965 -> [w1988]
          tunnel: [w1988] -> w1964
          tunnel: w1964 -> [w1989]
          tunnel: [w1989] -> w1966
          tunnel: w1966 -> [w1995]
          frame #0 {
            n1292 = property on="Save ave N" class="DigNum (strict)"("Val(Sgnl)"="Save ave factor") -> ()  [unwired: 2 in, 2 out]
          }
          frame #1 {
            n1293 = Wait (ms)(milliseconds to wait=u32 100) -> ()  [unwired: 1 out]
          }
          frame #2 {
            n1294 = local read "Offset 2 Start (MHz)"() -> (w1980:dbl)
            n1295 = property on="Saved AOD Raster Scan Parameter Sets" class="Arr (strict)"("Index Values"=u32[] [2]) -> ()  [unwired: 2 in, 2 out]
            n1296 = property on="Trap Delta (MHz)" class="DigNum (strict)"("Val(Sgnl)"=w1980) -> ()  [unwired: 2 in, 2 out]
          }
          frame #3 {
            n1297 = property on="Load parameters" class="Bool (strict)"("Val(Sgnl)"=TRUE ("Value (Signaling)")) -> ()  [unwired: 2 in, 2 out]
          }
          frame #4 {
            n1298 = Wait (ms)(milliseconds to wait=u32 100) -> ()  [unwired: 1 out]
          }
          frame #5 {
            n1299 = property on="Trap Raster Scan" class="Bool (strict)"("Val(Sgnl)"=TRUE ("Value (Signaling)")) -> ()  [unwired: 2 in, 2 out]
          }
          frame #6 {
            n1300 = Wait (ms)(milliseconds to wait=u32 1000) -> ()  [unwired: 1 out]
          }
          frame #7 {
            n1301 = while {
              stop <- w1992 stop-if-true
              n1302 = local read "Raster Scanning..."() -> (w1994:bool)
              n1303 = local read "Saving..."() -> (w1993:bool)
              n1304 = Not(x=w1993) -> (.not. x?=w1990:bool)
              n1305 = Not(x=w1994) -> (.not. x?=w1991:bool)
              n1306 = And(x=w1991, y=w1990) -> (x .and. y?=w1992:bool)
            }
          }
          frame #8 {
            n1307 = property on="Save ave N" class="DigNum (strict)"("Val(Sgnl)"=w1995) -> ()  [unwired: 2 in, 2 out]
          }
        }
      }
      event "Step Size (nm)": Value Change {
        n1308 = event-data() -> ()  [unwired: 1 in, 5 out]
        n1309 = flat-sequence {
          frame #0 {
            n1310 = property on="Saved AOD Raster Scan Parameter Sets" class="Arr (strict)"("Index Values"=u32[] [1]) -> ()  [unwired: 2 in, 2 out]
          }
          frame #1 {
            n1311 = Multiply(x="N Steps", y="Step Size (nm)") -> (x*y=w1997:dbl)
            n1312 = property on="Scan Speed AOD (nm/s) 2" class="DigNum (strict)"("Value"="Step Size (nm)") -> ()  [unwired: 2 in, 2 out]
            n1313 = property on="Step Size AOD (nm) 2" class="DigNum (strict)"("Value"="Step Size (nm)") -> ()  [unwired: 2 in, 2 out]
            n1314 = property on="Scan Range AOD (nm) 2" class="DigNum (strict)"("Value"=w1997) -> ()  [unwired: 2 in, 2 out]
          }
        }
      }
      event "Take Detection Laser\nImage": Value Change {
        n1315 = event-data() -> ()  [unwired: 1 in, 5 out]
        n1316 = flat-sequence {
          tunnel: [w2025] -> w2015
          tunnel: [w2024] -> w2008
          tunnel: [w2023] -> w2000
          tunnel: [w2028] -> w2016
          tunnel: w2015 -> [w2028]
          tunnel: [w2027] -> w2009
          tunnel: w2008 -> [w2027]
          tunnel: [w2026] -> w2001
          tunnel: w2000 -> [w2026]
          tunnel: [w2032] -> w2017
          tunnel: w2016 -> [w2032]
          tunnel: [w2031] -> w2010
          tunnel: w2009 -> [w2031]
          tunnel: [w2030] -> w2002
          tunnel: w2001 -> [w2030]
          tunnel: [w2038] -> w2018
          tunnel: w2017 -> [w2038]
          tunnel: [w2037] -> w2011
          tunnel: w2010 -> [w2037]
          tunnel: [w2036] -> w2003
          tunnel: w2002 -> [w2036]
          tunnel: [w2042] -> w2019
          tunnel: w2018 -> [w2042]
          tunnel: [w2041] -> w2012
          tunnel: w2011 -> [w2041]
          tunnel: [w2040] -> w2004
          tunnel: w2003 -> [w2040]
          tunnel: [w2046] -> w2020
          tunnel: w2019 -> [w2046]
          tunnel: [w2045] -> w2013
          tunnel: w2012 -> [w2045]
          tunnel: [w2044] -> w2005
          tunnel: w2004 -> [w2044]
          tunnel: [w2050] -> w2021
          tunnel: w2020 -> [w2050]
          tunnel: [w2049] -> w2014
          tunnel: w2013 -> [w2049]
          tunnel: [w2048] -> w2006
          tunnel: w2005 -> [w2048]
          tunnel: w2021 -> [w2056]
          tunnel: w2014 -> [w2055]
          tunnel: [w2053] -> w2007
          tunnel: w2006 -> [w2053]
          tunnel: w2007 -> [w2057]
          frame #0 {
            n1317 = local read "Green Laser ON/Interlacing"() -> (w2025:bool)
            n1318 = local read "Green laser mode"() -> (w2024:enum32{"Laser ON", "Laser OFF", "Interlace"})
            n1319 = local read "Green FB On/Off"() -> (w2023:bool)
          }
          frame #1 {
            n1320 = property on="Green FB On/Off" class="Bool (strict)"("Val(Sgnl)"=FALSE ("Value (Signaling)")) -> ()  [unwired: 2 in, 2 out]
          }
          frame #2 {
            n1321 = property on="Green Laser ON/Interlacing" class="Bool (strict)"("Val(Sgnl)"=TRUE ("Value (Signaling)")) -> ()  [unwired: 2 in, 2 out]
            n1322 = property on="Flip Green Filter" class="Bool (strict)"("Val(Sgnl)"=TRUE ("Value (Signaling)")) -> ()  [unwired: 2 in, 2 out]
            n1323 = property on="Green laser mode" class="RadioBtnsControl (strict)"("Val(Sgnl)"=enum32{"Laser ON", "Laser OFF", "Interlace"}."Laser ON" ("Value (Signaling)")) -> ()  [unwired: 2 in, 2 out]
          }
          frame #3 {
            n1324 = Wait (ms)(milliseconds to wait=u32 500) -> ()  [unwired: 1 out]
          }
          frame #4 {
            n1325 = property on="Confocal Image" class="Bool (strict)"("Val(Sgnl)"=TRUE ("Value (Signaling)")) -> ()  [unwired: 2 in, 2 out]
          }
          frame #5 {
            n1326 = Wait (ms)(milliseconds to wait=u32 2000) -> ()  [unwired: 1 out]
          }
          frame #6 {
            n1327 = while {
              stop <- w2051 stop-if-true
              n1328 = local read "Saving..."() -> (w2052:bool)
              n1329 = Not(x=w2052) -> (.not. x?=w2051:bool)
            }
          }
          frame #7 {
            n1330 = property on="Flip Green Filter" class="Bool (strict)"("Val(Sgnl)"=TRUE ("Value (Signaling)")) -> ()  [unwired: 2 in, 2 out]
            n1331 = property on="Green Laser ON/Interlacing" class="Bool (strict)"("Val(Sgnl)"=w2056) -> ()  [unwired: 2 in, 2 out]
            n1332 = property on="Green laser mode" class="RadioBtnsControl (strict)"("Val(Sgnl)"=w2055) -> ()  [unwired: 2 in, 2 out]
          }
          frame #8 {
            n1333 = property on="Green FB On/Off" class="Bool (strict)"("Val(Sgnl)"=w2057) -> ()  [unwired: 2 in, 2 out]
          }
        }
      }
      event "Stop All": Value Change {
        n1334 = event-data() -> ()  [unwired: 1 in, 5 out]
        n1335 = local read "Stop All"() -> (w2058:bool)
      }
    }
    n1336 = node-c288() -> ()  [unwired: 1 in, 1 out]
  }
  n1337 = node-c288() -> (w111:T25)  [unwired: 4 out]
  n1338 = timed-loop "Mouse control: trap position (AOM deflection), set confocal spot from image" {
    tunnel: [w2060] -> w71
    tunnel: w62 -> [w2059]
    timing: w111 -> [_]
    timing-out: [_] -> w110
    stop <- w2060 stop-if-true
    n1339 = node-c288() -> ()  [unwired: 2 out]
    n1340 = event shown="[0] \"Pane\": Mouse Down" {
      selector: _ -> [_ _]
      dyn-events: _ -> [_ _]
      timeout: _ -> [_ _]
      tunnel: w2059 -> [w2063 _]
      event Mouse Down {
        n1341 = event-data() -> ("Time"=w2065:u32, "Coords"=w2064:T8, "Button"=w2066:u16)  [unwired: 6 out]
        n1342 = case shown="1" w2066 {
          tunnel: w2065 -> [_ _ w2169]
          tunnel: w2064 -> [_ w2103 w2167]
          tunnel: w2063 -> [_ _ w2165]
          frame 0, Default {
          }
          frame 1 {
            n1343 = property on="APD 2"() -> ("Displayed Image Size"=w2072)  [unwired: 2 in, 2 out]
            n1344 = property on="APD 1"() -> ("Displayed Image Size"=w2100)  [unwired: 2 in, 2 out]
            n1345 = property on="Detection Laser X"() -> ("Displayed Image Size"=w2101)  [unwired: 2 in, 2 out]
            n1346 = property on="Detection Laser Y"() -> ("Displayed Image Size"=w2097)  [unwired: 2 in, 2 out]
            n1347 = property on="APD 2"() -> ("Displayed Image Position"=w2073)  [unwired: 2 in, 2 out]
            n1348 = property on="APD 1"() -> ("Displayed Image Position"=w2102)  [unwired: 2 in, 2 out]
            n1349 = property on="Detection Laser X"() -> ("Displayed Image Position"=w2099)  [unwired: 2 in, 2 out]
            n1350 = property on="Detection Laser Y"() -> ("Displayed Image Position"=w2098)  [unwired: 2 in, 2 out]
            n1351 = Unbundle By Name(w2072) -> ("Width"=w2069, "Height"=w2068)
            n1352 = Unbundle By Name(w2073) -> ("Left"=w2071, "Top"=w2070)
            n1353 = Unbundle By Name(w2100) -> ("Width"=w2094, "Height"=w2093)
            n1354 = Unbundle By Name(w2101) -> ("Width"=w2090, "Height"=w2089)
            n1355 = Unbundle By Name(w2097) -> ("Width"=w2086, "Height"=w2085)
            n1356 = Unbundle By Name(w2102) -> ("Left"=w2096, "Top"=w2095)
            n1357 = Unbundle By Name(w2099) -> ("Left"=w2092, "Top"=w2091)
            n1358 = Unbundle By Name(w2098) -> ("Left"=w2088, "Top"=w2087)
            n1359 = Bundle("Left"=w2071, "Top"=w2070, "Width"=w2069, "Height"=w2068) -> (w2067:T34)  [unwired: 1 in]
            n1360 = Bundle("Left"=w2096, "Top"=w2095, "Width"=w2094, "Height"=w2093) -> (w2084:T34)  [unwired: 1 in]
            n1361 = Bundle("Left"=w2092, "Top"=w2091, "Width"=w2090, "Height"=w2089) -> (w2083:T34)  [unwired: 1 in]
            n1362 = Bundle("Left"=w2088, "Top"=w2087, "Width"=w2086, "Height"=w2085) -> (w2082:T34)  [unwired: 1 in]
            n1363 = Build Cluster Array(w2067, w2084, w2083, w2082) -> (w2081:T35)
            n1364 = for {
              tunnel: w2103 -> [w2114]
              tunnel: w2081 -> [w2115] mode=indexing
              shift-right: [w2112] -> w2079
              shift-left: TRUE -> [w2113]
              shift-right: [w2111] -> w2077
              shift-left: _ -> [w2107]
              shift-right: [w2110] -> w2076
              shift-left: _ -> [w2106]
              shift-right: [w2109] -> w2075
              shift-left: _ -> [w2105]
              shift-right: [w2108] -> w2074
              shift-left: _ -> [w2104]
              n1365 = case shown="True" w2113 {
                selector: w2113 -> [w2120 _]
                tunnel: w2115 -> [_ w2129]
                tunnel: w2114 -> [_ w2127]
                tunnel: [w2120 w2125] -> w2112
                tunnel: [w2119 w2124] -> w2111
                tunnel: [w2118 w2123] -> w2110
                tunnel: [w2117 w2122] -> w2109
                tunnel: [w2116 w2121] -> w2108
                tunnel: w2107 -> [w2119 _]
                tunnel: w2106 -> [w2118 _]
                tunnel: w2105 -> [w2117 _]
                tunnel: w2104 -> [w2116 _]
                frame False {
                }
                frame True {
                  n1366 = Unbundle(w2129) -> (w2128:T34)
                  n1367 = call "isclickinwindow.vi"("Image Param"=w2128, "Point32"=w2127) -> ("Y px"=w2121:i32, "Height"=w2122:i32, "X px"=w2123:i32, "Width"=w2124:i32, "In image?"=w2126:bool)  [unwired: 1 in]
                  n1368 = Not(x=w2126) -> (.not. x?=w2125:bool)
                }
              }
            }
            n1369 = Not(x=w2079) -> (.not. x?=w2078:bool)
            n1370 = case shown="True" w2078 {
              tunnel: w2076 -> [_ w2142]
              tunnel: w2074 -> [_ w2141]
              tunnel: w2077 -> [_ w2140]
              tunnel: w2075 -> [_ w2139]
              frame False {
              }
              frame True {
                w2135 = FALSE ("Get Point")
                n1371 = local read "Scan lines (y)"() -> (w2144:u64)
                n1372 = local read "Actual MCL Inc (V)"() -> (w2136:dbl)
                n1373 = local read "Scan steps (MCL)"() -> (w2143:u64)
                n1374 = Divide "Y Pix/step"(x=w2139, y=w2144) -> (x/y=w2151:dbl)
